vi "Magnet Limits.vi"(0 "instrument.PPMS":refnum<class "instrument.PPMS.lvclass">, 5 "Helium (%)":dbl, 7 "Target Field (Oe)":dbl, 9 "Mode":T1, 11 "error in (no error)":errorcluster) -> (4 "instrument.PPMS out":refnum<class "instrument.PPMS.lvclass">, 8 "Limited Field (Oe)":dbl, 10 "Mode out":T1, 15 "error out":errorcluster)   [LabVIEW 2019, in "instrument.PPMS.lvclass"]
uses:
  instrument.PPMS.lvclass
  <userlib>/LevyLab/Instrument Framework/Instrument Types/Cryostat/Typedefs/Magnet Mode--Enum.ctl
  <userlib>/LevyLab/Instrument Framework/Instrument Types/Cryostat/Instrument.Cryostat.lvclass
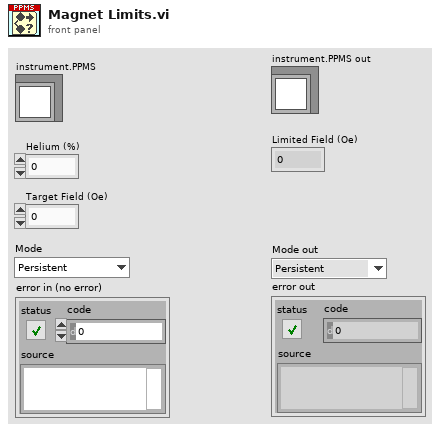
[diagram p1: front panel]
types:
  T1 = typedef "Instrument.Cryostat.lvclass/Magnet Mode--Enum.ctl" = enum16{"Persistent", "Driven"}
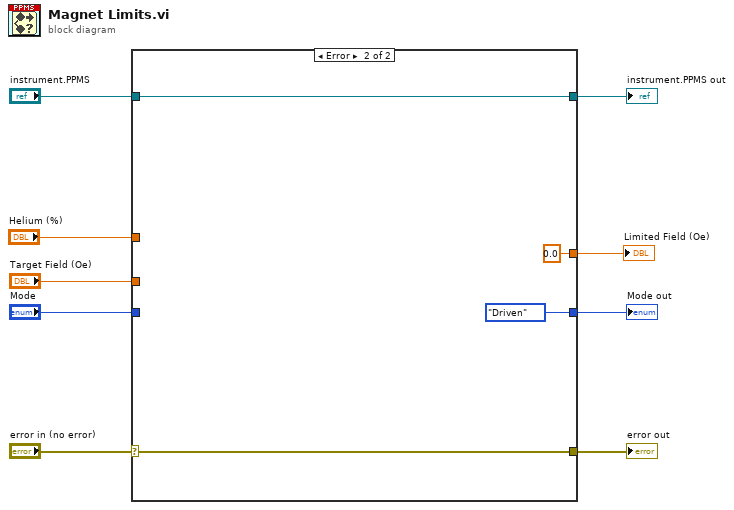
[diagram p0: block diagram]
diagram:
  n1 = case shown="Error" "error in (no error)" {
    selector: "error in (no error)" -> [w12 w17]
    tunnel: "Target Field (Oe)" -> [w10 _]
    tunnel: [w10 0.0 ("upper limit")] -> w8
    tunnel: "instrument.PPMS" -> [w13 w16]
    tunnel: [w13 w16] -> w6
    tunnel: [w12 w17] -> w5
    tunnel: "Helium (%)" -> [_ _]
    tunnel: [w11 Magnet_Mode--Enum."Driven" ("Mode")] -> w2
    tunnel: "Mode" -> [w11 _]
    frame No Error {
    }
    frame Error {
    }
  }
  "Limited Field (Oe)" <- w8
  "instrument.PPMS out" <- w6
  "Mode out" <- w2
  "error out" <- w5
